vi "Send Update VI Title.vi"(7 "Message Priority (Normal)":T1=enum."Normal", 8 "error in (no error)":errorcluster, 10 "New Title":string, 11 "Message Enqueuer":refnum<class "Message Enqueuer.lvclass">) -> (0 "error out":errorcluster, 3 "Message Enqueuer out":refnum<class "Message Enqueuer.lvclass">)   [LabVIEW 2020, in "Chat Window UI Controller.lvlib" / "Update VI Title Msg.lvclass"]
doc: "This VI sends the message to an actor."
uses:
  Update VI Title Msg.lvclass
  <vilib>/ActorFramework/Message Enqueuer/Message Enqueuer.lvclass
  <vilib>/ActorFramework/Message Enqueuer/Message Priority.ctl
  C:/Program Files (x86)/National Instruments/LabVIEW 2020/vi.lib/ActorFramework/Message/Message.lvclass
  Update VI Title Msg.lvclass/Update VI Title Msg.ctl
  <vilib>/ActorFramework/Message Enqueuer/Message Enqueuer.lvclass/Message Enqueuer.ctl
  <vilib>/ActorFramework/Message Priority Queue/Priority Enqueue.vi
  F:/Gitlab Repository/LabVIEW-Study/10.Top 5 Actor Framework Overrides/Chat Room with Interface/Chat Window UI Controller/Chat Window UI Controller Messages/Update VI Title Msg/Update VI Title Msg.lvclass
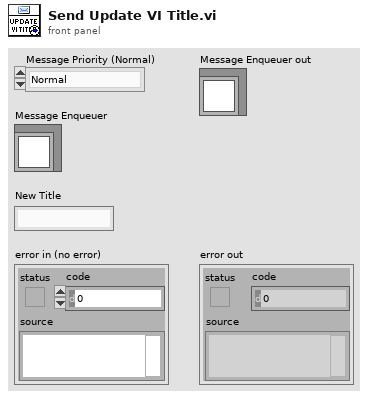
[diagram p1: front panel]
types:
  T1 = typedef "Actor Framework.lvlib/Message Enqueuer.lvclass/Message Priority.ctl" = enum16{"Low", "Normal", "High"}
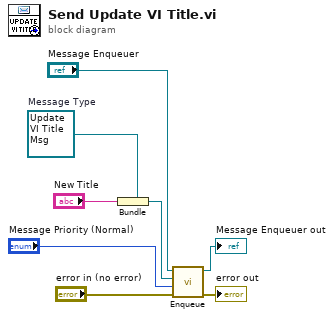
[diagram p0: block diagram]
diagram:
  w5 = refnum<class "Update VI Title Msg.lvclass"> refnum  # Message Type
  n1 = Bundle(cluster=w5, "New Title") -> (w4:refnum<class "Update VI Title Msg.lvclass">)
  n2 = call <vilib>:"Enqueue.vi"("error in (no error)"="error in (no error)", "Message Priority (Normal)"="Message Priority (Normal)", "Message"=w4, "Message Enqueuer in"="Message Enqueuer") -> ("error out"=→"error out":errorcluster, "Message Enqueuer in"=→"Message Enqueuer out":refnum<class "Message Enqueuer.lvclass">)  [unwired: 6 in]
